vi "Lab2_AMdemodulation.vi"() -> ()   [LabVIEW 2010]
uses:
  <vilib>/measure/maspectr.llb/FFT Spectrum (Mag-Phase) for N Chan.vi
  <vilib>/measure/NI_MAPro.lvlib
  <vilib>/measure/NI_MABase.lvlib
  <vilib>/ptbypt/NI_PtbyPt.lvlib
  <vilib>/Analysis/NI_AALPro.lvlib
panel:
  out "DC estimate (V)":dbl format="%0.2f"
  out "Demodulated/AM\n(DSB-SC)":dbl
  out "Demodulated/AM\n(Conventional DSB)":dbl
  out "DSB-SC Demodulated (time)\nSynchronous Demodulation":dynamicdata(graph)
  out "DSB-SC Demodulated (frequency)\nSynchronous Demodulation":cluster{"f0":dbl, "df":dbl, "magnitude":dbl[]}[](graph)
  out "DSB-SC Baseband (frequency)":cluster{"f0":dbl, "df":dbl, "magnitude":dbl[]}(graph)
  out "DSB-SC Baseband (time)":waveform(dbl)(graph)
  in  "phase":dbl
  in  "stop":bool
  out "Conventional Demodulated (frequency)\nEnvelop Detector":cluster{"f0":dbl, "df":dbl, "magnitude":dbl[]}[](graph)
  out "Conventional Demodulated (time)\nEnvelop Detector":dynamicdata(graph)
  out "Conventional Baseband (time)":waveform(dbl)(graph)
  out "Conventional Baseband (frequency)":cluster{"f0":dbl, "df":dbl, "magnitude":dbl[]}(graph)
  in  "baseband amplitude":dbl(slide)=1.0 scale=0.0..2.0
  in  "mod index":dbl(slide)=1.0 scale=0.0..1.0
  in  "modulation frequency":dbl(knob)=10.0 scale=0.0..1000.0
  in  "carrier frequency":dbl(knob)=10.0 scale=0.0..500000.0
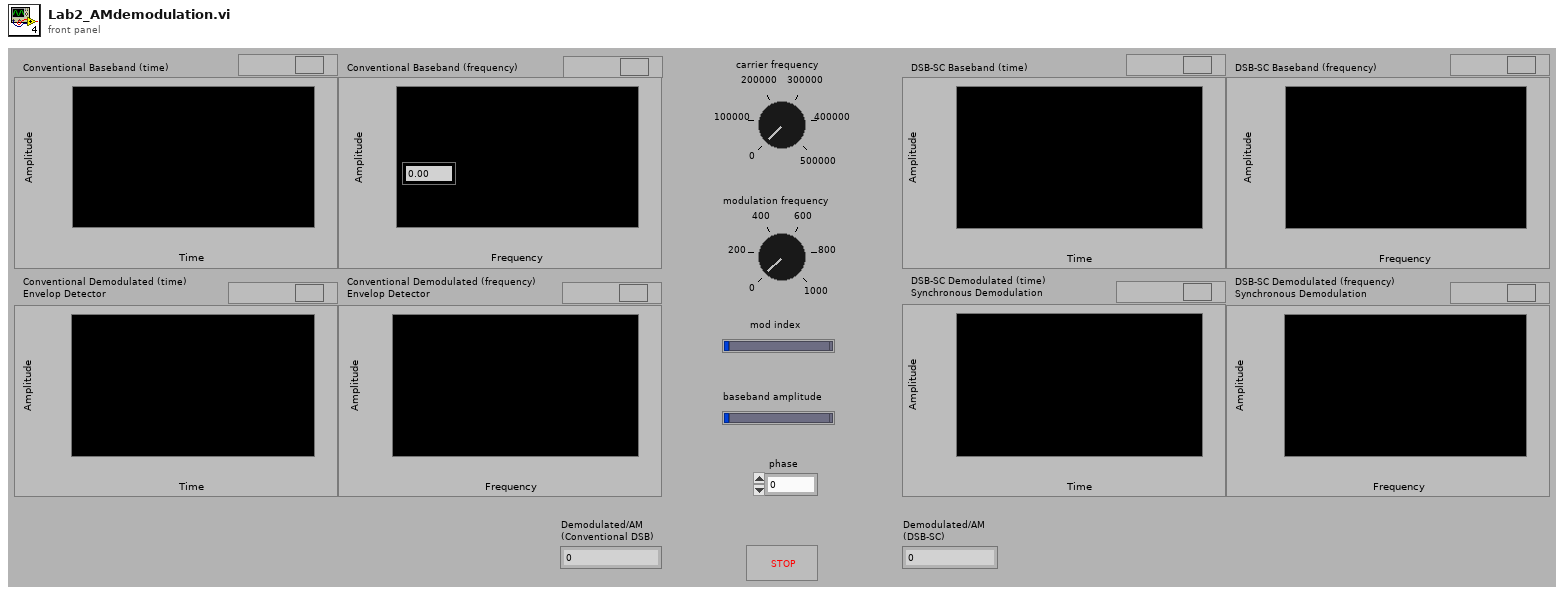
[diagram p1: front panel]
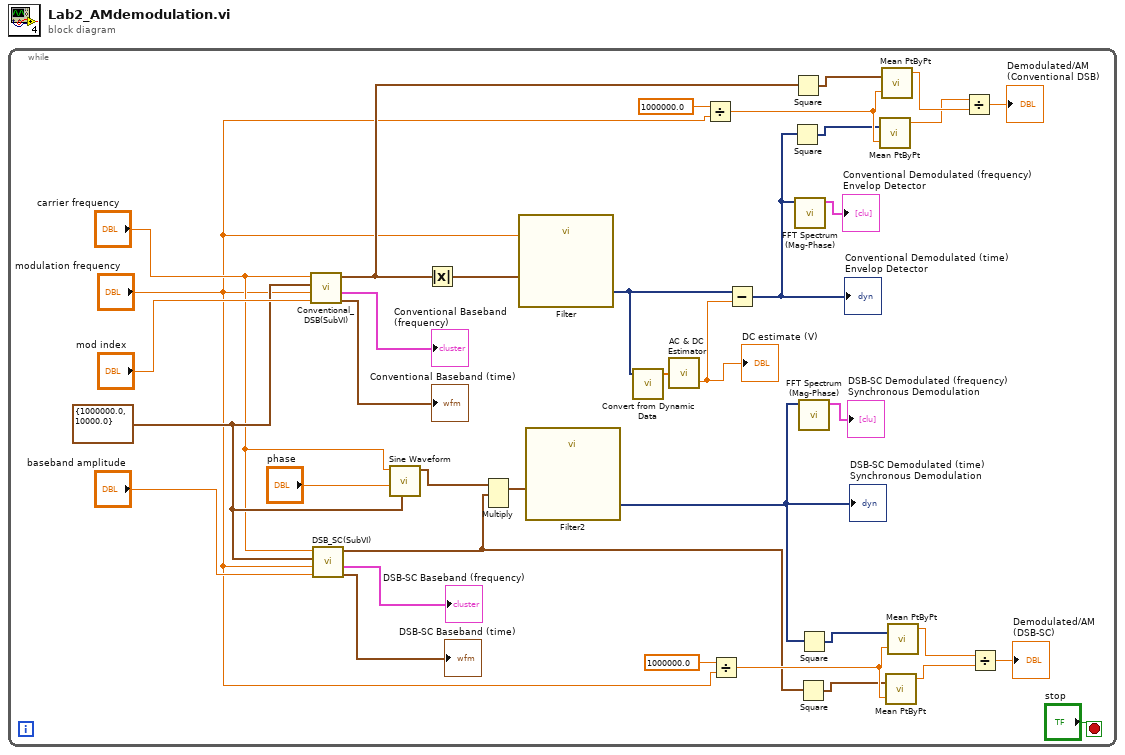
[diagram p0: block diagram]
diagram:
  n1 = while {
    stop <- "stop" stop-if-true
    w30 = cluster{"Fs":dbl, "#s":dbl} {"Fs"=1000000.0, "#s"=10000.0} ("sampling info")
    n2 = call "Conventional_DSB(SubVI).vi"("mod index"="mod index", "modulation frequency"="modulation frequency", "sampling info"=w30, "carrier frequency"="carrier frequency") -> ("baseband signal (time-domain)"=→"Conventional Baseband (time)":waveform(dbl), "baseband signal (frequency-domain)"=→"Conventional Baseband (frequency)":cluster{"f0":dbl, "df":dbl, "magnitude":dbl[]}, "modulated signal (time-domain)"=w15:waveform(dbl))  [unwired: 1 out]
    n3 = call "DSB_SC(SubVI).vi"("message amplitude"="baseband amplitude", "modulation frequency"="modulation frequency", "sampling info"=w30, "carrier frequency"="carrier frequency") -> ("baseband signal (time-domain)"=→"DSB-SC Baseband (time)":waveform(dbl), "baseband signal (frequency-domain)"=→"DSB-SC Baseband (frequency)":cluster{"f0":dbl, "df":dbl, "magnitude":dbl[]}, "modulated signal (time-domain)"=w6:waveform(dbl))  [unwired: 1 out]
    n4 = call <vilib>:"Sine Waveform.vi"("sampling info"=w30, "phase"="phase", "frequency"="carrier frequency") -> ("signal out"=w25:waveform(dbl))  [unwired: 7 in, 1 out]
    n5 = Absolute Value(x=w15) -> (abs(x)=w29:waveform(dbl))
    n6 = Multiply(1:w6, 2:w25) -> (0:w26:waveform(dbl))  [unwired: 1 in, 1 out]
    n7 = call "Filter"("Lower Cut-Off"="modulation frequency", "Signal"=w29) -> ("Filtered Signal"=w2:dynamicdata)  [unwired: 8 in, 1 out]
    n8 = call "Filter2"("Signal"=w26) -> ("Filtered Signal"=w7:dynamicdata)  [unwired: 9 in, 1 out]
    "DSB-SC Demodulated (time)\nSynchronous Demodulation" <- w7
    n9 = call "Convert from Dynamic Data"("Dynamic Data Type"=w2) -> ("Array"=w3:dbl[])  [unwired: 3 in]
    n10 = call <vilib>:"AC & DC Estimator.vi"("Signal (V)"=w3) -> ("DC estimate (V)"=w1:dbl)  [unwired: 1 out]
    "DC estimate (V)" <- w1
    n11 = Divide(x=1000000.0, y="modulation frequency") -> (x/y=w19:dbl)
    n12 = Divide(x=1000000.0, y="modulation frequency") -> (x/y=w12:dbl)
    n13 = Subtract(x=w2, y=w1) -> (x-y=w14:dynamicdata)
    "Conventional Demodulated (time)\nEnvelop Detector" <- w14
    n14 = Square(x=w14) -> (x^2=w16:dynamicdata)
    n15 = Square(x=w15) -> (x^2=w17:waveform(dbl))
    n16 = call-poly <vilib>:"FFT Spectrum (Mag-Phase).vi"("time signals"=w14) -> ("magnitudes"=→"Conventional Demodulated (frequency)\nEnvelop Detector":cluster{"f0":dbl, "df":dbl, "magnitude":dbl[]}[])  [unwired: 6 in, 4 out]
    n17 = Square(x=w6) -> (x^2=w9:waveform(dbl))
    n18 = call-poly <vilib>:"FFT Spectrum (Mag-Phase).vi"("time signals"=w7) -> ("magnitudes"=→"DSB-SC Demodulated (frequency)\nSynchronous Demodulation":cluster{"f0":dbl, "df":dbl, "magnitude":dbl[]}[])  [unwired: 6 in, 4 out]
    n19 = Square(x=w7) -> (x^2=w10:dynamicdata)
    n20 = call <vilib>:"Mean PtByPt.vi"("x"=w16, "sample length"=w19) -> ("mean"=w21:dbl)  [unwired: 2 in, 1 out]
    n21 = call <vilib>:"Mean PtByPt.vi"("x"=w17, "sample length"=w19) -> ("mean"=w22:dbl)  [unwired: 2 in, 1 out]
    n22 = call <vilib>:"Mean PtByPt.vi"("x"=w9, "sample length"=w12) -> ("mean"=w4:dbl)  [unwired: 2 in, 1 out]
    n23 = call <vilib>:"Mean PtByPt.vi"("x"=w10, "sample length"=w12) -> ("mean"=w5:dbl)  [unwired: 2 in, 1 out]
    n24 = Divide(x=w21, y=w22) -> (x/y=→"Demodulated/AM\n(Conventional DSB)":dbl)
    n25 = Divide(x=w5, y=w4) -> (x/y=→"Demodulated/AM\n(DSB-SC)":dbl)
  }
